vi "XYToMotorValue.vi"(8 "Y":dbl, 11 "X":dbl) -> (0 "Right":dbl, 3 "Left":dbl)   [LabVIEW 2014]
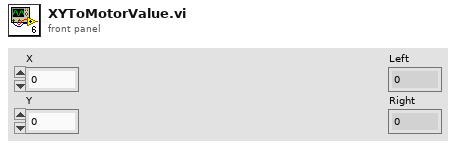
[diagram p1: front panel]
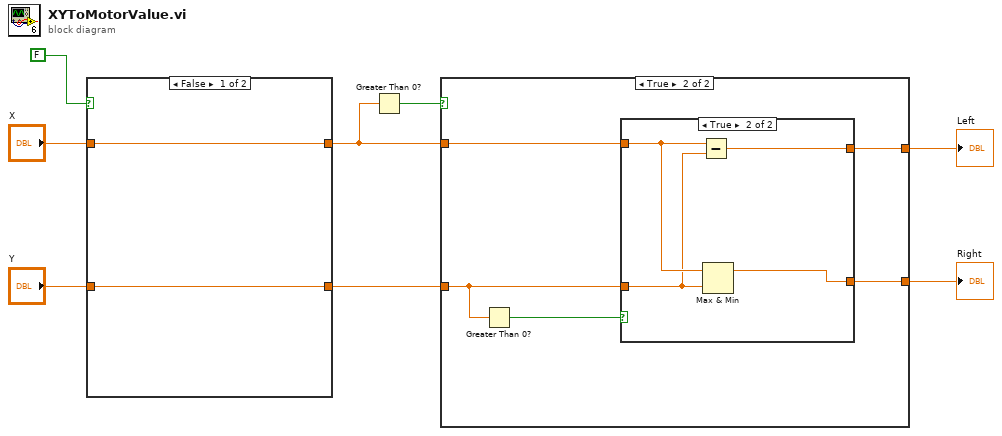
[diagram p0: block diagram]
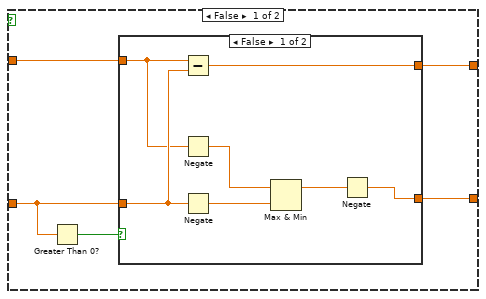
[diagram p2: hidden frame]
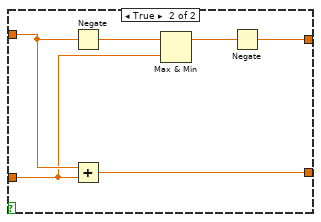
[diagram p3: hidden frame]
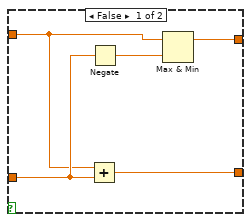
[diagram p4: hidden frame]
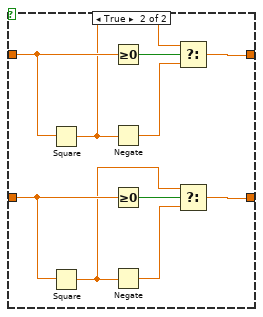
[diagram p5: hidden frame]
diagram:
  n1 = case shown="False" FALSE {
    tunnel: [w9 w20] -> w6
    tunnel: [w10 w19] -> w7
    tunnel: "Y" -> [w9 w18]
    tunnel: "X" -> [w10 w17]
    frame False {
    }
    frame True {
      n2 = Square(x=w17) -> (x^2=w12:dbl)
      n3 = Square(x=w18) -> (x^2=w15:dbl)
      n4 = Greater Or Equal To 0?(x=w17) -> (x >= 0?=w11:bool)
      n5 = Negate(x=w12) -> (-x=w13:dbl)
      n6 = Greater Or Equal To 0?(x=w18) -> (x >= 0?=w16:bool)
      n7 = Negate(x=w15) -> (-x=w14:dbl)
      n8 = Select(t=w12, s=w11, f=w13) -> (s? t:f=w19:dbl)
      n9 = Select(t=w15, s=w16, f=w14) -> (s? t:f=w20:dbl)
    }
  }
  n10 = Greater Than 0?(x=w7) -> (x > 0?=w8:bool)
  n11 = case shown="True" w8 {
    tunnel: w6 -> [w24 w42]
    tunnel: w7 -> [w23 w41]
    tunnel: [w22 w40] -> w2
    tunnel: [w21 w39] -> w1
    frame False {
      n12 = Greater Than 0?(x=w24) -> (x > 0?=w25:bool)
      n13 = case shown="False" w25 {
        tunnel: w24 -> [w32 w34]
        tunnel: w23 -> [w30 w35]
        tunnel: [w26 w36] -> w22
        tunnel: [w27 w33] -> w21
        frame False {
          n14 = Subtract(x=w30, y=w32) -> (x-y=w26:dbl)
          n15 = Negate(x=w30) -> (-x=w31:dbl)
          n16 = Negate(x=w32) -> (-x=w29:dbl)
          n17 = Max & Min(x=w31, y=w29) -> (max(x,y)=w28:dbl)  [unwired: 1 out]
          n18 = Negate(x=w28) -> (-x=w27:dbl)
        }
        frame True {
          n19 = Negate(x=w35) -> (-x=w38:dbl)
          n20 = Add(x=w35, y=w34) -> (x+y=w33:dbl)
          n21 = Max & Min(x=w38, y=w34) -> (max(x,y)=w37:dbl)  [unwired: 1 out]
          n22 = Negate(x=w37) -> (-x=w36:dbl)
        }
      }
    }
    frame True {
      n23 = Greater Than 0?(x=w42) -> (x > 0?=w43:bool)
      n24 = case shown="True" w43 {
        tunnel: w42 -> [w48 w50]
        tunnel: w41 -> [w45 w51]
        tunnel: [w46 w49] -> w40
        tunnel: [w44 w52] -> w39
        frame False {
          n25 = Add(x=w45, y=w48) -> (x+y=w44:dbl)
          n26 = Negate(x=w48) -> (-x=w47:dbl)
          n27 = Max & Min(x=w45, y=w47) -> (max(x,y)=w46:dbl)  [unwired: 1 out]
        }
        frame True {
          n28 = Subtract(x=w51, y=w50) -> (x-y=w49:dbl)
          n29 = Max & Min(x=w51, y=w50) -> (max(x,y)=w52:dbl)  [unwired: 1 out]
        }
      }
    }
  }
  "Left" <- w2
  "Right" <- w1
